vi "Do.vi"(8 "error in (no error)":errorcluster, 10 "Actor in":refnum<class "Actor.lvclass">, 11 "StartImageAcquisition Msg":refnum<class "StartImageAcquisition Msg.lvclass">) -> (0 "error out":errorcluster, 2 "Actor out":refnum<class "Actor.lvclass">)   [LabVIEW 2020, in "StartImageAcquisition Msg.lvclass"]
doc: "This VI delivers the message to the actor by calling the appropriate method(s) on the actor."
uses:
  StartImageAcquisition Msg.lvclass
  <vilib>/ActorFramework/Actor/Actor.lvclass
  StartImageAcquisition Msg.lvclass/StartImageAcquisition Msg.ctl
  MicroscopeIO/MicroscopeIO.lvclass
  9ef47adc-f318-494c-9b8b-6df3216d6863.vi
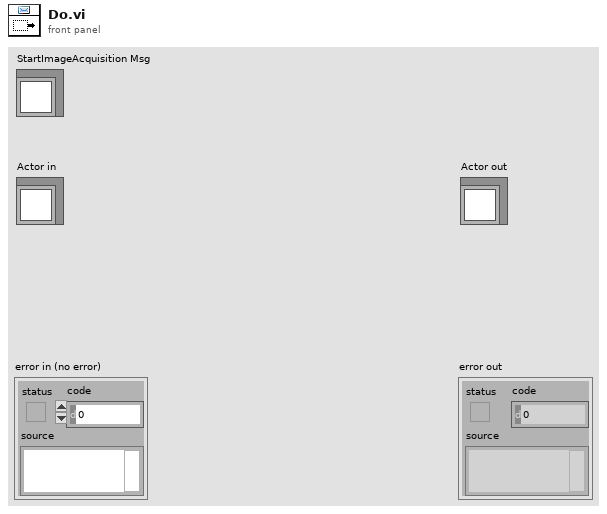
[diagram p1: front panel]
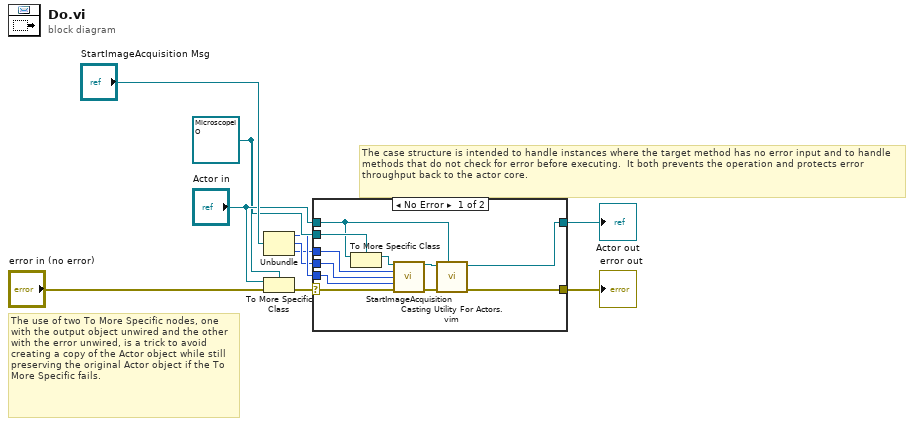
[diagram p0: block diagram]
diagram:
  w4 = refnum<class "MicroscopeIO.lvclass"> refnum ("Actor in")
  # "The use of two To More Specific nodes, one with the output object unwired and the other with the error unwired, is a trick to avoid creating a copy of the Actor object while still preserving the original Actor object if the To More Specific fails."
  # "The case structure is intended to handle instances where the target method has no error input and to handle methods that do not check for error before executing.  It both prevents the operation and protects error throughput back to the actor core."
  n1 = Unbundle("StartImageAcquisition Msg") -> (w3:i32, w2:i32, w1:i32)
  n2 = To More Specific Class(target class=w4, reference="Actor in", error in="error in (no error)") -> (error out=w8:errorcluster)  [unwired: 1 out]
  n3 = case shown="No Error" w8 {
    selector: w8 -> [w21 w23]
    tunnel: [w15 w23] -> w7
    tunnel: [w16 w22] -> w6
    tunnel: "Actor in" -> [w18 w22]
    tunnel: w4 -> [w19 _]
    tunnel: w3 -> [w13 _]
    tunnel: w2 -> [w12 _]
    tunnel: w1 -> [w11 _]
    frame No Error {
      n4 = To More Specific Class(target class=w19, reference=w18) -> (specific class reference=w20:refnum<class "MicroscopeIO.lvclass">)  [unwired: 1 in, 1 out]
      n5 = call-dynamic "StartImageAcquisition.vi"("Communication in"=w20, "Exposure"=w11, "Frames"=w12, "Interval"=w13, "error in (no error)"=w21) -> ("Communication out"=w17:refnum<class "MicroscopeIO.lvclass">, "error out"=w14:errorcluster)  [unwired: 9 in]
      n6 = call "Casting Utility For Actors.vim"("type"=w18, "error in (no error)"=w14, "Actor in"=w17) -> ("error out"=w15:errorcluster, "Actor out"=w16:refnum<class "Actor.lvclass">)  [unwired: 7 in]
    }
    frame Error {
      # "If type check fails, pass the original object out again."
    }
  }
  "error out" <- w7
  "Actor out" <- w6
